vi "Populate Existing Channels.vi"(8 "error in (no error)":errorcluster, 9 "Parent Tag":string, 10 "Shared Variable Channel Info":T1 {"Channel Refs" format="%.0x"}, 11 "TreeControl in":refnum<vi>) -> (0 "error out":errorcluster, 3 "TreeControl out":refnum<vi>)   [LabVIEW 2015, in "Shared Variable Custom Device.lvlib"]
uses:
  Shared Variable Custom Device.lvlib
  Engine/Support/Channel Information Control.ctl
  <vilib>/NI Veristand/Custom Device API/Custom Device Item Ref.ctl
  <vilib>/Utility/VariantDataType/Type.ctl
  <vilib>/NI Veristand/Custom Device API/Custom Device API.lvlib
  <vilib>/Utility/VariantDataType/VariantType.lvlib
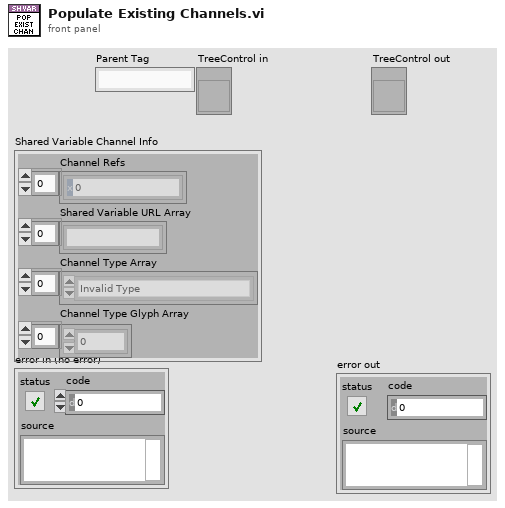
[diagram p1: front panel]
types:
  T1 = typedef "Shared Variable Custom Device.lvlib/Channel Information Control.ctl" = cluster{"Channel Refs":T2[], "Shared Variable URL Array":string[], "Channel Type Array":T3[], "Channel Type Glyph Array":i32[]}
  T2 = typedef "Custom Device API.lvlib/Custom Device Item Ref.ctl" = u64
  T3 = typedef "VariantType.lvlib/Type.ctl" = enum8{"Invalid Type", "Void", "I8", "I16", "I32", "I64", "U8", "U16", "U32", "U64", "Single Float", "Double Float", "Extended Float", "Single Complex", "Double Complex", "Extended Complex", "Enum U8", "Enum U16", "Enum U32", "Enum U64", "Single Float With Unit", "Double Float With Unit", "Extended Float With Unit", "Single Complex with Unit", "Double Complex with Unit", "Extended Complex with Unit", "Boolean", "String", "Path", "Picture", "Tag", "Array", "Cluster", "Variant", "LV Variant", "Waveform", "Timestamp", "Digital Waveform", "Digital Data", "ExpressData", "Refnum", "External Data", "VI", "Poly VI", "LabVIEW Class Instance", "Fixed Point"}
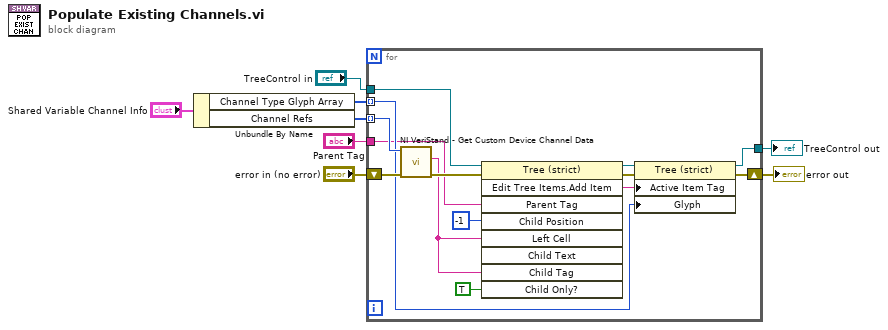
[diagram p0: block diagram]
diagram:
  n1 = Unbundle By Name("Shared Variable Channel Info") -> ("Channel Type Glyph Array"=w8:i32[], "Channel Refs"=w7:T2[])
  n2 = for {
    tunnel: "TreeControl in" -> [w19]
    tunnel: w7 -> [w22] mode=indexing
    tunnel: w8 -> [w15] mode=indexing
    tunnel: [w14] -> w1
    shift-right: [w13] -> w4
    shift-left: "error in (no error)" -> [w21]
    tunnel: "Parent Tag" -> [w9]
    n3 = call <vilib>:"NI VeriStand - Get Custom Device Channel Data.vi"("error in (no error)"=w21, "Channel Ref in"=w22) -> ("error out"=w20:errorcluster, "Channel Name"=w11:string)  [unwired: 4 in, 4 out]
    n4 = invoke on="Invoke Node" class="Tree (strict)" method="Edit Tree Items.Add Item"(reference=w19, error in=w20, "Parent Tag"=w9, "Child Position"=-1, "Left Cell"=w11, "Child Tag"=w11, "Child Only?"=TRUE) -> (reference out=w17:refnum<vi>, error out=w18:errorcluster, "Edit Tree Items:Add Item"=w16:string)  [unwired: 2 in, 6 out]
    n5 = property on="Property Node" class="Tree (strict)"(reference=w17, error in=w18, "Active Item Tag"=w16, "Glyph"=w15) -> (reference out=w14:refnum<vi>, error out=w13:errorcluster)
  }
  "error out" <- w4
  "TreeControl out" <- w1
